vi "MSSQL Example.vi"() -> ()   [LabVIEW 2020]
uses:
  <vilib>/Viviota/shared/ORM_ADONet.lvlibp/ADOMapper/ADOMapper.lvclass
  C:/Program Files/National Instruments/LabVIEW 2020/vi.lib/Viviota/shared/ORM.lvlibp/ORM/SqlMapper/SqlMapper.lvclass
  ORM_API/ORM_API.lvlib
  7567ee1f-f747-46f7-b4dd-0c9fb0e63776.vi
  AlbumMap/AlbumMap.lvclass
  Album/Album.lvclass
  df564c15-4522-450c-b99f-f01b994daeb7.vi
  C:/Program Files/National Instruments/LabVIEW 2020/vi.lib/Viviota/shared/ORM_ADONet.lvlibp/ADOMapper/ADOMapper.lvclass
  <vilib>/Viviota/shared/ORM_DBC_Mssql.lvlibp/SQL Connect.vi
  <vilib>/Viviota/shared/ORM_DBC_Mssql.lvlibp/DBC.lvclass
panel:
  out "error out":errorcluster
  out "id":variant
  out "Title 2":string
  out "Primary Key":i64
  in  "Title":string
  out "Value":variant
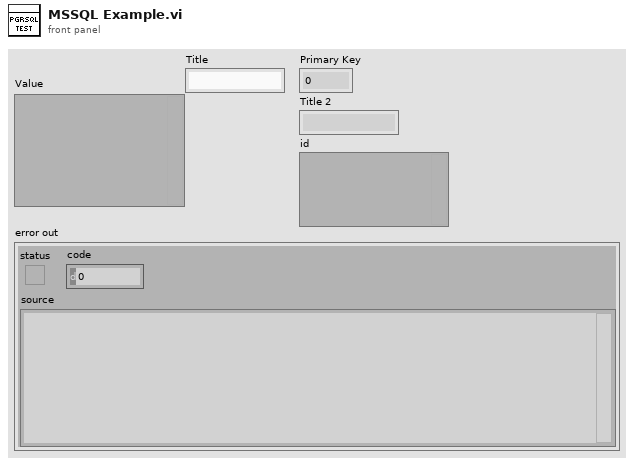
[diagram p1: front panel]
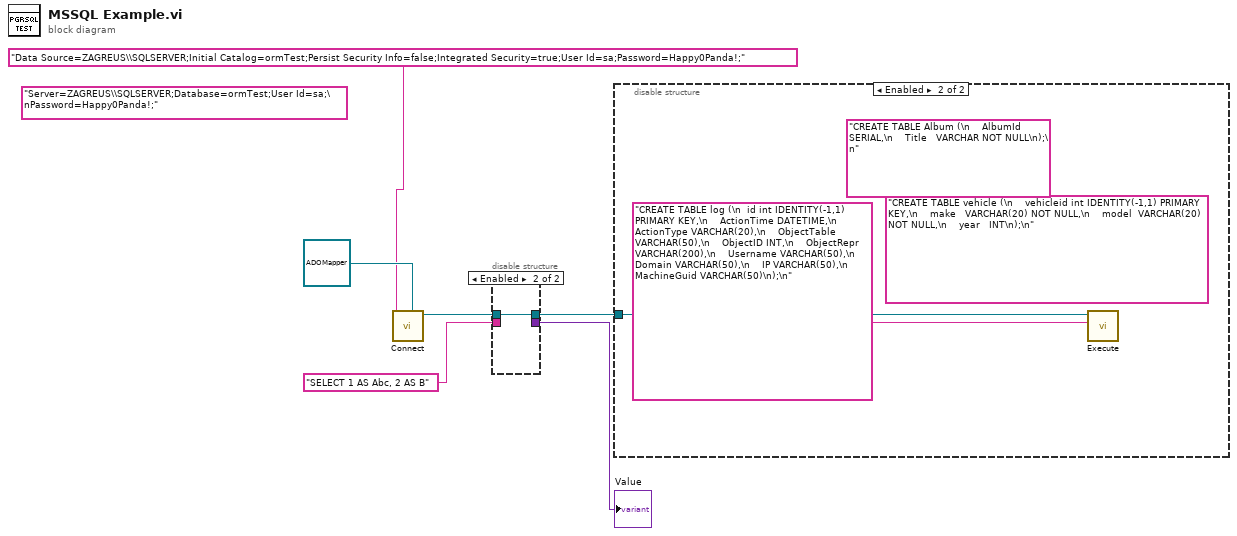
[diagram p0: block diagram]
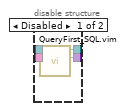
[diagram p2: hidden frame]
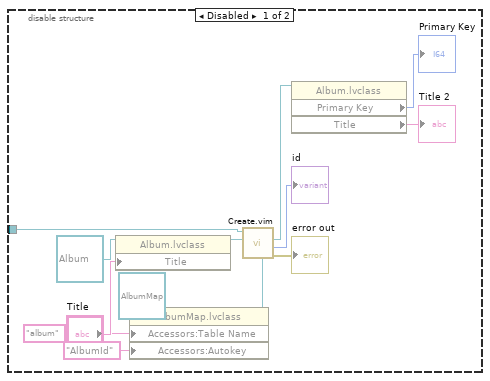
[diagram p3: hidden frame]
diagram:
  (unwired) "Server=ZAGREUS\\SQLSERVER;Database=ormTest;User Id=sa;\nPassword=Happy0Panda!;"
  n1 = call-poly "Connect.vi"("SqlMapper Type"=refnum<class "ADOMapper.lvclass"> refnum ("ADONet.lvlib:ADOMapper.lvclass"), "Connection String"="Data Source=ZAGREUS\\SQLSERVER;Initial Catalog=ormTest;Persist Security Info=false;Integrated Security=true;User Id=sa;Password=Happy0Panda!;") -> ("SQL Mapper"=w6:refnum<class "ADOMapper.lvclass">)  [unwired: 8 in, 1 out]
  n2 = disable-structure shown="Enabled" {
    disable-tunnel: w6 -> [w10 w11]
    disable-tunnel: "SELECT 1 AS Abc, 2 AS B" ("sql") -> [w9 _]
    disable-tunnel: [w8 _] -> w4
    disable-tunnel: [w7 w11] -> w3
    frame Disabled {
      n3 = call "QueryFirst_SQL.vim"("sql"=w9, "SqlMapper in"=w10) -> ("Value"=w8:refnum<class>, "SqlMapper out"=w7:refnum<class "ADOMapper.lvclass">)  [unwired: 7 in, 1 out]
    }
    frame Enabled {
    }
  }
  "Value" <- w4
  n4 = disable-structure shown="Enabled" {
    disable-tunnel: w3 -> [w24 w26]
    frame Disabled {
      n5 = property class="Album.lvclass"(reference=refnum<class "Album.lvclass"> refnum ("Album.lvclass"), "Title"="Title") -> (reference out=w20:refnum<class "Album.lvclass">)  [unwired: 1 in, 1 out]
      n6 = property class="AlbumMap.lvclass"(reference=refnum<class "AlbumMap.lvclass"> refnum ("AlbumMap.lvclass"), "Accessors:Table Name"="album" ("Log Table Name"), "Accessors:Autokey"="AlbumId" ("Autokey")) -> (reference out=w14:refnum<class "AlbumMap.lvclass">)  [unwired: 1 in, 1 out]
      n7 = call "Create.vim"("TypeMap in"=w14, "object in"=w20, "SqlMapper in"=w24) -> ("error out"=→"error out":errorcluster, "id"=→"id":i32, "object out"=w19:refnum<class "Album.lvclass">)  [unwired: 5 in, 1 out]
      n8 = property class="Album.lvclass"(reference=w19) -> ("Primary Key"=→"Primary Key":i64, "Title"=→"Title 2":string)  [unwired: 1 in, 2 out]
    }
    frame Enabled {
      (unwired) "CREATE TABLE vehicle (\n    vehicleid int IDENTITY(-1,1) PRIMARY KEY,\n    make   VARCHAR(20) NOT NULL,\n    model  VARCHAR(20) NOT NULL,\n    year   INT\n);\n" ("sql")
      (unwired) "CREATE TABLE Album (\n    AlbumId SERIAL,\n    Title   VARCHAR NOT NULL\n);\n" ("sql")
      n9 = call-dynamic "Execute.vi"("sql"="CREATE TABLE log (\n  id int IDENTITY(-1,1) PRIMARY KEY,\n    ActionTime DATETIME,\n    ActionType VARCHAR(20),\n    ObjectTable VARCHAR(50),\n    ObjectID INT,\n    ObjectRepr VARCHAR(200),\n    Username VARCHAR(50),\n    Domain VARCHAR(50),\n    IP VARCHAR(50),\n    MachineGuid VARCHAR(50)\n);\n", "ADOMapper in"=w26) -> ()  [unwired: 7 in, 3 out]
    }
  }
